vi "Lake Shore Cryotronics 370 Application AC Resistance Bridge.vi"() -> ()   [LabVIEW 2012]
doc: "This VI was designed to demonstrate typical usage of sub vi's containing the more common 370 functions.\n\nThis example configures the control parameters and setpoint of the instrument, allows for a delay, and then reads sensor and heater output data. The user is given the option of just reading data and not configuring the instrument."
uses:
  <instrlib>/Lake Shore Cryotronics 370/Lake Shore Cryotronics 370.lvlib
panel:
  in  "VISA resource name":refnum<visa-resource-name>
  out "Heater Output":dbl(slide) min=0.0 max=100.0 step=1e-05 scale=0.0..100.0 scale format="%^.2e"
  out "Power Reading":dbl min=0.0 max=0.01 step=1e-05 format="%^.5e"
  out "Kelvin Reading":dbl min=0.0 max=1000.0 step=1e-05 format="%^.5e"
  in  "Channel (1)":i32=1 min=1 max=16 step=1
  out "Resistance Reading":dbl min=0.0 max=63200000.0 step=1e-05 format="%^.5e"
  in  "Setpoint (0.00000E+0)":dbl min=0.0 max=100000000.0 step=1e-06 format="%^.5e"
  in  "Heater Range (0: Off)":u16(ring) items=["Off", "31.6 uA", "100 uA", "316 uA", "1.00 mA", "3.16 mA", "10.0 mA", "31.6 mA", "100 mA"]
  in  "Manual Output (0.000)":dbl min=0.0 max=100.0 step=0.001 format="%.3f"
  in  "Rate (D) (0)":dbl min=0.0 max=2500.0 step=1.0
  in  "Reset (I) (20)":dbl=20.0 min=0.0 max=10000.0 step=1.0
  in  "Gain (P) (10.000)":dbl=10.0 min=0.001 max=1000.0 step=0.001 format="%.3f"
  in  "Configure (False)":bool
  # "(c) 2001 - 2009 National Instruments.  ALL RIGHTS RESERVED."
  # "%"
  # "370 AC Resistance Bridge"
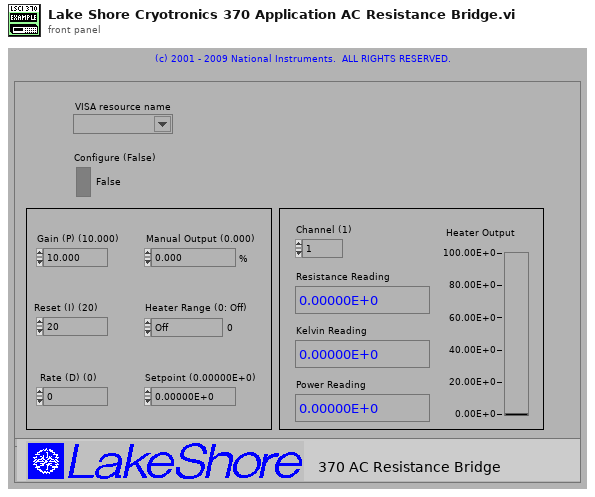
[diagram p1: front panel]
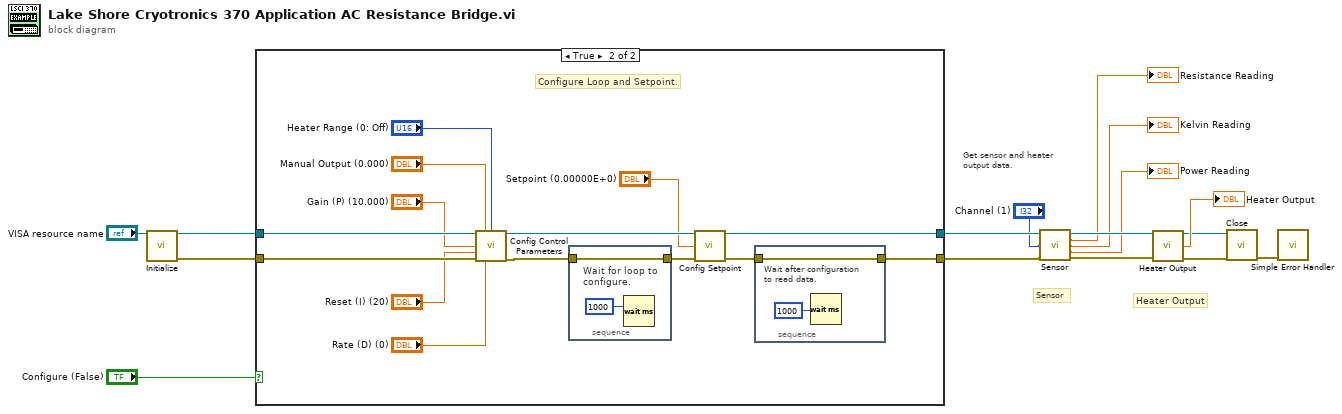
[diagram p0: block diagram]
diagram:
  # "Heater Output"
  # "Sensor"
  # "Get sensor and heater\noutput data."
  n1 = call <instrlib>:"Initialize.vi"("VISA resource name"="VISA resource name") -> ("VISA resource name out"=w14:refnum<visa-resource-name>, "error out"=w15:errorcluster)  [unwired: 13 in]
  n2 = case shown="True" "Configure (False)" {
    tunnel: w15 -> [w17 w30]
    tunnel: w14 -> [w18 w29]
    tunnel: [w17 w32] -> w11
    tunnel: [w18 w20] -> w12
    frame False {
      # "Do not configure Loop and Setpoint."
    }
    frame True {
      # "Configure Loop and Setpoint."
      n3 = call <instrlib>:"Config Control Parameters.vi"("VISA resource name"=w29, "Manual Output (0.000%)"="Manual Output (0.000)", "Heater Range (0: Off)"="Heater Range (0: Off)", "Gain(P) (10.000)"="Gain (P) (10.000)", "Reset(I) (20)"="Reset (I) (20)", "error in (no error)"=w30, "Rate(D) (0)"="Rate (D) (0)") -> ("VISA resource name out"=w21:refnum<visa-resource-name>, "error out"=w31:errorcluster)  [unwired: 7 in]
      n4 = stacked-sequence {
        tunnel: w31 -> [w35]
        tunnel: [w35] -> w23
        frame #0 {
          # "Wait for loop to \nconfigure."
          n5 = Wait (ms)(milliseconds to wait=u32 1000) -> ()  [unwired: 1 out]
        }
      }
      n6 = call <instrlib>:"Config Setpoint.vi"("VISA resource name"=w21, "Setpoint (0.00000E+0)"="Setpoint (0.00000E+0)", "error in (no error)"=w23) -> ("VISA resource name out"=w20:refnum<visa-resource-name>, "error out"=w22:errorcluster)  [unwired: 11 in]
      n7 = stacked-sequence {
        tunnel: w22 -> [w34]
        tunnel: [w34] -> w32
        frame #0 {
          # "Wait after configuration\nto read data."
          n8 = Wait (ms)(milliseconds to wait=1000) -> ()  [unwired: 1 out]
        }
      }
    }
  }
  n9 = call <instrlib>:"Sensor.vi"("VISA resource name"=w12, "Channel (1)"="Channel (1)", "error in (no error)"=w11) -> ("VISA resource name out"=w8:refnum<visa-resource-name>, "Resistance Reading"=→"Resistance Reading":dbl, "Kelvin Reading"=→"Kelvin Reading":dbl, "Power Reading"=→"Power Reading":dbl, "error out"=w9:errorcluster)  [unwired: 8 in]
  n10 = call <instrlib>:"Heater Output.vi"("VISA resource name"=w8, "error in (no error)"=w9) -> ("VISA resource name out"=w3:refnum<visa-resource-name>, "Heater Output"=→"Heater Output":dbl, "error out"=w4:errorcluster)  [unwired: 11 in]
  n11 = call <instrlib>:"Close.vi"("VISA resource name"=w3, "error in (no error)"=w4) -> ("error out"=w2:errorcluster)  [unwired: 13 in]
  n12 = call <vilib>:"Simple Error Handler.vi"("error in (no error)"=w2) -> ()  [unwired: 4 in, 5 out]
